vi "cmd RandGen.vi"(8 "error in (no error)":errorcluster, 11 "Controller in":refnum<class "Controller.lvclass">) -> (0 "error out":errorcluster, 3 "Controller out":refnum<class "Controller.lvclass">)   [LabVIEW 2020, in "Controller.lvlib" / "Controller.lvclass"]
uses:
  Controller.lvclass
  Controller.lvclass/Controller.ctl
  Actor_log/Actor_log Messages/Write Event to Log Msg/Write Event to Log Msg.lvclass/Write Event to Log Msg.ctl
  <vilib>/ActorFramework/Message Enqueuer/Message Enqueuer.lvclass/Message Enqueuer.ctl
  <vilib>/ActorFramework/Message Enqueuer/Enqueue.vi
  Actor_log/Actor_log Messages/Write Event to Log Msg/Write Event to Log Msg.lvclass
  C:/Program Files/National Instruments/LabVIEW 2020/vi.lib/ActorFramework/Message/Message.lvclass
  <vilib>/ActorFramework/Message Priority Queue/Priority Enqueue.vi
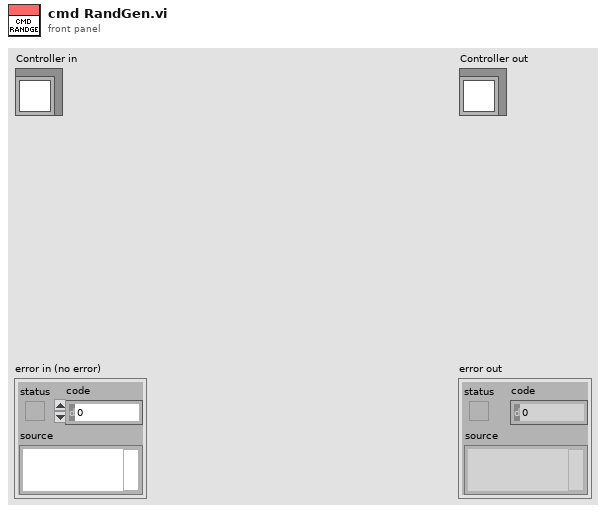
[diagram p1: front panel]
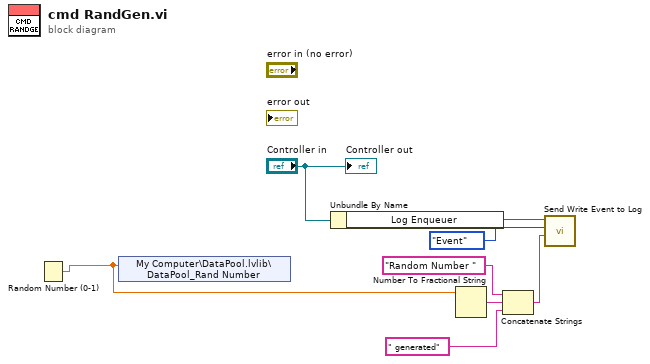
[diagram p0: block diagram]
diagram:
  n1 = Random Number (0-1)() -> (number: 0 to 1=w5:dbl)
  n2 = shared-variable "My Computer\\DataPool.lvlib\\DataPool_Rand Number"(w5) -> ()  [unwired: 1 in, 1 out]
  n3 = Unbundle By Name("Controller in") -> ("Log Enqueuer"=w7:refnum<class "Message Enqueuer.lvclass">)
  n4 = Number To Fractional String(number=w5) -> (F-format string=w4:string)  [unwired: 3 in]
  n5 = Concatenate Strings("Random Number ", w4, " generated") -> (w1:string)
  n6 = call "Send Write Event to Log.vi"("Log Event Details"=w1, "Enum"=enum16{"Event", "Error"}."Event", "Message Enqueuer"=w7) -> ()  [unwired: 7 in, 2 out]
  "Controller out" <- "Controller in"
